vi "LDR.vi"() -> ()   [LabVIEW 2022 SP3]
uses:
  <vilib>/DAQmx/read.llb/DAQmx Read (Analog DBL 1Chan 1Samp).vi
  <vilib>/DAQmx/write.llb/DAQmx Write (Digital Bool 1Line 1Point).vi
  <vilib>/DAQmx/create/channels.llb/DAQmx Create Channel (AI-Voltage-Basic).vi
  <vilib>/DAQmx/create/channels.llb/DAQmx Create Channel (DO-Digital Output).vi
  <vilib>/DAQmx/miscellaneous.llb/DAQmx Fill In Error Info.vi
panel:
  in  "lines 2":tag
  in  "lines":tag
  in  "stop 2":bool
  out "Intensity Indicator":dbl(knob) scale=0.0..1000.0
  out "Measurement":dbl(knob) scale=0.0..2.0
  in  "stop":bool
  in  "physical channels":tag
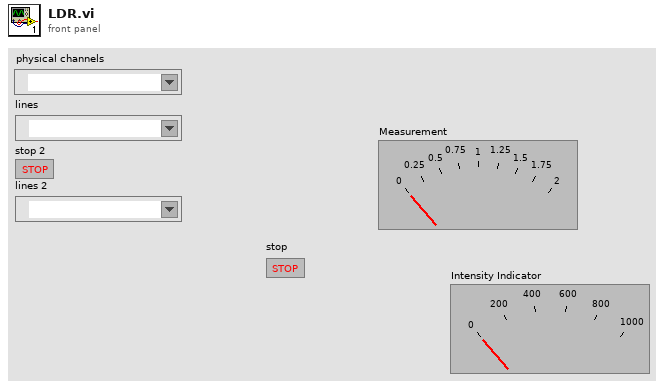
[diagram p1: front panel]
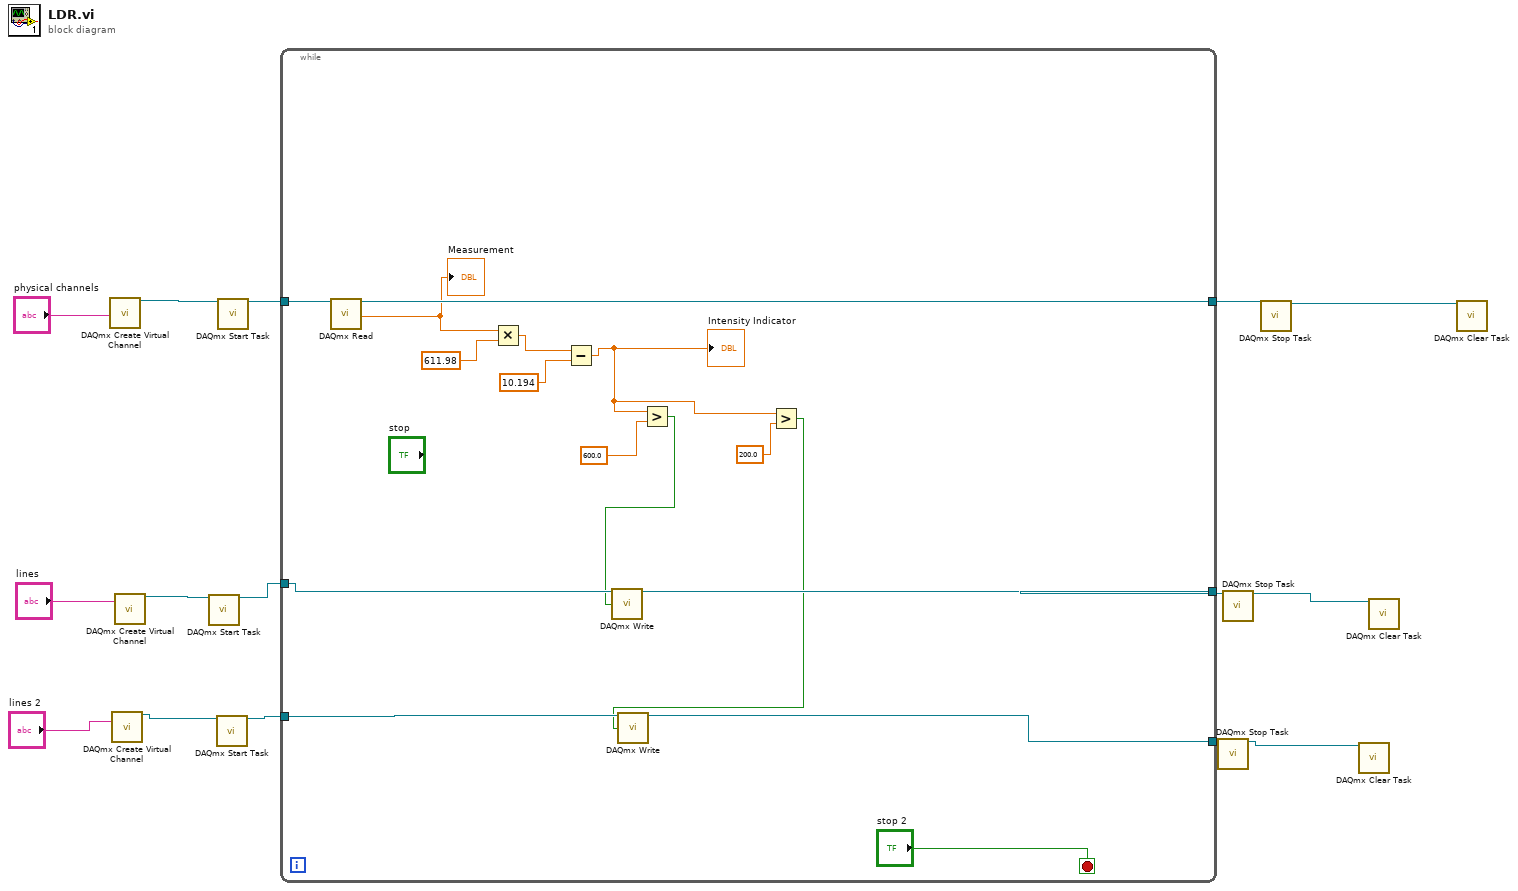
[diagram p0: block diagram]
diagram:
  n1 = call-poly <vilib>:"DAQmx Create Virtual Channel.vi"("physical channels"="physical channels") -> ("task out"=w14:refnum<k21>)  [unwired: 13 in, 1 out]
  n2 = call-poly <vilib>:"DAQmx Create Virtual Channel.vi"("lines"="lines 2") -> ("task out"=w4:refnum<k21>)  [unwired: 13 in, 1 out]
  n3 = call-poly <vilib>:"DAQmx Create Virtual Channel.vi"("lines"="lines") -> ("task out"=w8:refnum<k21>)  [unwired: 13 in, 1 out]
  n4 = call <vilib>:"DAQmx Start Task.vi"("task/channels in"=w8) -> ("task out"=w10:refnum<k21>)  [unwired: 13 in, 1 out]
  n5 = call <vilib>:"DAQmx Start Task.vi"("task/channels in"=w4) -> ("task out"=w3:refnum<k21>)  [unwired: 13 in, 1 out]
  n6 = call <vilib>:"DAQmx Start Task.vi"("task/channels in"=w14) -> ("task out"=w13:refnum<k21>)  [unwired: 13 in, 1 out]
  n7 = while {
    tunnel: w13 -> [w31]
    tunnel: [w30] -> w11
    tunnel: w10 -> [w26]
    tunnel: [w23] -> w6
    tunnel: w3 -> [w20]
    tunnel: [w19] -> w2
    stop <- "stop 2" stop-if-true
    n8 = call-poly <vilib>:"DAQmx Read.vi"("task/channels in"=w31) -> ("task out"=w30:refnum<k21>, "data"=w29:dbl)  [unwired: 12 in, 1 out]
    "Measurement" <- w29
    n9 = Multiply(x=w29, y=611.98) -> (x*y=w22:dbl)
    n10 = Subtract(x=w22, y=10.194) -> (x-y=w17:dbl)
    "Intensity Indicator" <- w17
    n11 = Greater?(x=w17, y=600.0) -> (0:w24:bool)
    n12 = call-poly <vilib>:"DAQmx Write.vi"("task/channels in"=w26, "data"=w24) -> ("task out"=w23:refnum<k21>)  [unwired: 11 in, 2 out]
    n13 = Greater?(x=w17, y=200.0) -> (0:w16:bool)
    n14 = call-poly <vilib>:"DAQmx Write.vi"("task/channels in"=w20, "data"=w16) -> ("task out"=w19:refnum<k21>)  [unwired: 11 in, 2 out]
  }
  n15 = call <vilib>:"DAQmx Stop Task.vi"("task/channels in"=w2) -> ("task out"=w1:refnum<k21>)  [unwired: 13 in, 1 out]
  n16 = call <vilib>:"DAQmx Stop Task.vi"("task/channels in"=w6) -> ("task out"=w9:refnum<k21>)  [unwired: 13 in, 1 out]
  n17 = call <vilib>:"DAQmx Stop Task.vi"("task/channels in"=w11) -> ("task out"=w12:refnum<k21>)  [unwired: 13 in, 1 out]
  n18 = call <vilib>:"DAQmx Clear Task.vi"("task in"=w1) -> ()  [unwired: 14 in, 1 out]
  n19 = call <vilib>:"DAQmx Clear Task.vi"("task in"=w9) -> ()  [unwired: 14 in, 1 out]
  n20 = call <vilib>:"DAQmx Clear Task.vi"("task in"=w12) -> ()  [unwired: 14 in, 1 out]
